vi "XControl with User Events Convert.vi"(2 "Container State":T1, 3 "Display State":T2) -> (1 "Display State To Save":variant)   [LabVIEW 2009, in "XControlUserEvents.xctl"]
doc: "Demonstration of an XControl.\n\nAAL 9/09"
uses:
  XControlUserEvents.xctl
  XControl with User Events State.ctl
  <vilib>/_xctls/Container State.ctl
  <vilib>/_xctls/XControlSupport.lvlib
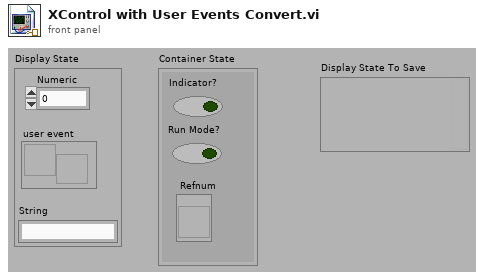
[diagram p1: front panel]
types:
  T1 = typedef "XControlSupport.lvlib/Container State.ctl" = cluster{"Indicator?":bool, "Run Mode?":bool, " Refnum":refnum<vi>}
  T2 = typedef "XControlUserEvents.xctl/XControl with User Events State.ctl" = cluster{"Numeric":dbl, "user event":refnum<user-event>, "String":string}
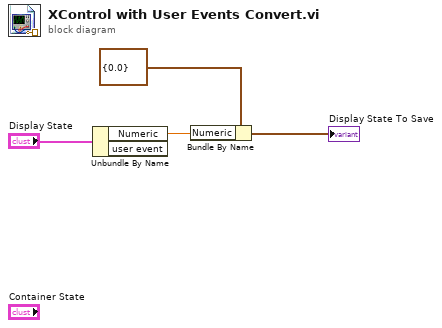
[diagram p0: block diagram]
diagram:
  n1 = Unbundle By Name("Display State") -> ("Numeric"=w2:dbl)  [unwired: 1 out]
  n2 = Bundle By Name(cluster=cluster{"Numeric":dbl} {"Numeric"=0.0}, "Numeric"=w2) -> (→"Display State To Save":cluster{"Numeric":dbl})
